vi "Creacion_array_inductivo.vi"() -> ()   [LabVIEW 2015]
panel:
  out "size(s)":i32
  out "Señal_digital":dbl[](array[numeric])
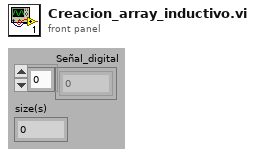
[diagram p1: front panel]
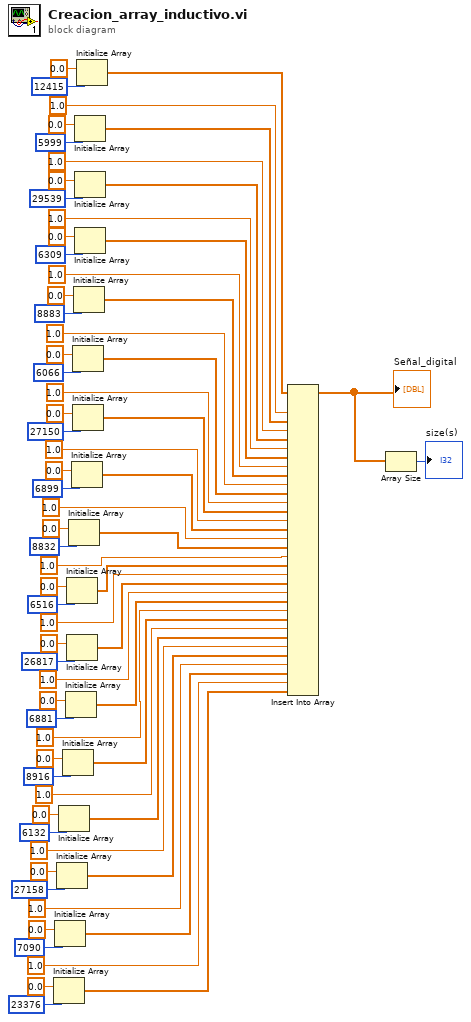
[diagram p0: block diagram]
diagram:
  n1 = Initialize Array(0.0 ("element"), 23376 ("dimension size")) -> (w1:dbl[])
  n2 = Initialize Array(0.0 ("element"), 7090 ("dimension size")) -> (w3:dbl[])
  n3 = Initialize Array(0.0 ("element"), 27158 ("dimension size")) -> (w5:dbl[])
  n4 = Initialize Array(0.0 ("element"), 6132 ("dimension size")) -> (w7:dbl[])
  n5 = Initialize Array(0.0 ("element"), 8916 ("dimension size")) -> (w9:dbl[])
  n6 = Initialize Array(0.0 ("element"), 6881 ("dimension size")) -> (w11:dbl[])
  n7 = Initialize Array(0.0 ("element"), 6516 ("dimension size")) -> (w15:dbl[])
  n8 = Initialize Array(0.0 ("element"), 26817 ("dimension size")) -> (w13:dbl[])
  n9 = Initialize Array(0.0 ("element"), 8832 ("dimension size")) -> (w17:dbl[])
  n10 = Initialize Array(0.0 ("element"), 6899 ("dimension size")) -> (w19:dbl[])
  n11 = Initialize Array(0.0 ("element"), 6066 ("dimension size")) -> (w23:dbl[])
  n12 = Initialize Array(0.0 ("element"), 27150 ("dimension size")) -> (w21:dbl[])
  n13 = Initialize Array(0.0 ("element"), 8883 ("dimension size")) -> (w25:dbl[])
  n14 = Initialize Array(0.0 ("element"), 5999 ("dimension size")) -> (w31:dbl[])
  n15 = Initialize Array(0.0 ("element"), 29539 ("dimension size")) -> (w29:dbl[])
  n16 = Initialize Array(0.0 ("element"), 6309 ("dimension size")) -> (w27:dbl[])
  n17 = Initialize Array(0.0 ("element"), 12415 ("dimension size")) -> (w35:dbl[])
  n18 = Insert Into Array(array=w35, new element #1=1.0 ("element"), new element #2=w31, new element #3=1.0 ("element"), new element #4=w29, new element #5=1.0 ("element"), new element #6=w27, new element #7=1.0 ("element"), new element #8=w25, new element #9=1.0 ("element"), new element #10=w23, new element #11=1.0 ("element"), new element #12=w21, new element #13=1.0 ("element"), new element #14=w19, new element #15=1.0 ("element"), new element #16=w17, new element #17=1.0 ("element"), new element #18=w15, new element #19=1.0 ("element"), new element #20=w13, new element #21=1.0 ("element"), new element #22=w11, new element #23=1.0 ("element"), new element #24=w9, new element #25=1.0 ("element"), new element #26=w7, new element #27=1.0 ("element"), new element #28=w5, new element #29=1.0 ("element"), new element #30=w3, new element #31=1.0 ("element"), new element #32=w1) -> (w34:dbl[])  [unwired: 1 in]
  "Señal_digital" <- w34
  n19 = Array Size(array=w34) -> (size(s)=→"size(s)":i32)
